vi "TDMS File Logging Test.vi"() -> ()   [LabVIEW 2021]
uses:
  <vilib>/Utility/sysdir.llb/System Directory Type.ctl
  <vilib>/Utility/TDMS File Viewer/NI_TDMS File Viewer.lvlib
panel:
  in  "View(F)":bool
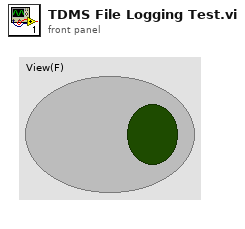
[diagram p1: front panel]
types:
  T1 = enum16{"open", "open or create", "create or replace", "create", "open (read-only)"}
  T2 = typedef "System Directory Type.ctl" = i32
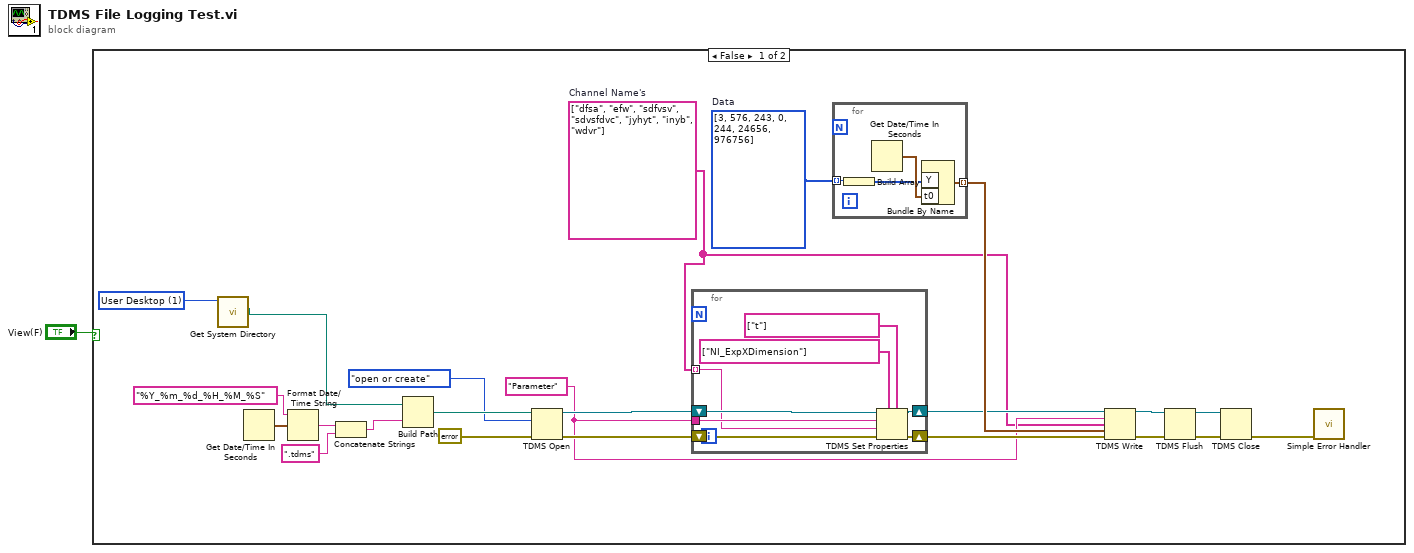
[diagram p0: block diagram]
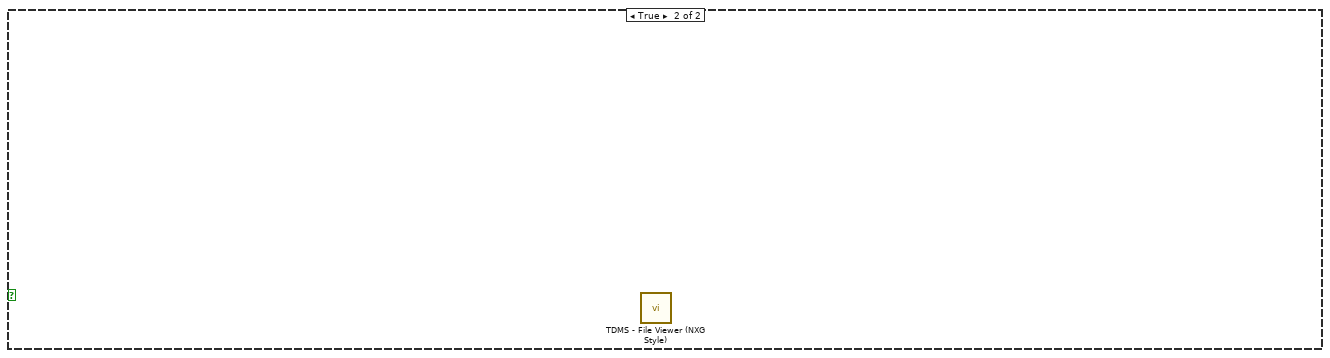
[diagram p2: hidden frame]
diagram:
  n1 = case shown="False" "View(F)" {
    frame False {
      w11 = T2 1 items=["User Home"=0, "User Desktop"=1, "User Documents"=2, "User Application Data"=3, "User Preferences"=4, "User Temporary"=5, "Public Documents"=6, "Public Application Data"=7, "Public Preferences"=8, "Public Cache"=13, "System Core Libraries"=9, "System Installed Libraries"=10, "Application Files"=11, "Boot Volume Root"=12] ("system directory type")
      w3 = "Parameter" ("group name in (Untitled)")
      w8 = i32[] [3, 576, 243, 0, 244, 24656, 976756]  # Data
      w2 = string[] ["dfsa", "efw", "sdfvsv", "sdvsfdvc", "jyhyt", "inyb", "wdvr"]  # Channel Name's
      n2 = call <vilib>:"Get System Directory.vi"("system directory type"=w11) -> ("system directory"=w10:path)  [unwired: 10 in]
      n3 = Get Date/Time In Seconds() -> (seconds since 1Jan1904=w24:timestamp)
      n4 = Format Date/Time String(time format string (%c)="%Y_%m_%d_%H_%M_%S", seconds (now)=w24) -> (date/time string=w23:string)  [unwired: 1 in]
      n5 = Concatenate Strings(w23, ".tdms" ("string")) -> (w20:string)
      n6 = Build Path(base path=w10, name or relative path=w20) -> (appended path=w19:path)
      n7 = TDMS Open(8:errorcluster {"status"=FALSE, "code"=0, "source"=""} ("error in (no error)"), 10:T1."open or create" ("operation (0:open)"), 11:w19) -> (0:w6:errorcluster, 3:w7:refnum<k34>)  [unwired: 4 in]
      n8 = for {
        tunnel: w3 -> [w27]
        shift-right: [w29] -> w5
        shift-left: w7 -> [w31]
        shift-right: [w28] -> w4
        shift-left: w6 -> [w30]
        tunnel: w2 -> [w25] mode=indexing
        n9 = TDMS Set Properties(5:string[] ["t"] ("property names"), 7:string[] ["NI_ExpXDimension"] ("property names"), 8:w30, 9:w25, 10:w27, 11:w31) -> (0:w28:errorcluster, 3:w29:refnum<k34>)  [unwired: 2 out]
      }
      n10 = for {
        tunnel: [w36] -> w9 mode=indexing
        tunnel: w8 -> [w34] mode=indexing
        n11 = Build Array(w34) -> (w33:i32[])
        n12 = Get Date/Time In Seconds() -> (seconds since 1Jan1904=w35:timestamp)
        n13 = Bundle By Name("Y"=w33, "t0"=w35) -> (w36:waveform(i32))  [unwired: 1 in]
      }
      n14 = TDMS Write(0:w5, 5:w3, 7:w2, 9:w9, 11:w4) -> (4:w15:refnum<k34>, 15:w16:errorcluster)  [unwired: 1 in, 2 out]
      n15 = TDMS Flush(4:w16, 7:w15) -> (0:w14:errorcluster, 3:w13:refnum<k34>)
      n16 = TDMS Close(8:w14, 11:w13) -> (0:w12:errorcluster)  [unwired: 1 out]
      n17 = call <vilib>:"Simple Error Handler.vi"("error in (no error)"=w12) -> ()  [unwired: 4 in, 5 out]
    }
    frame True {
      n18 = call <vilib>:"TDMS - File Viewer (NXG Style).vi"() -> ()  [unwired: 10 in, 2 out]
    }
  }
